vi "enumerateStaticDependencies.vi"(8 "error in (no error)":errorcluster, 11 "SMO.Example":refnum<class "SMO.TopLevel.lvclass">) -> (0 "error out":errorcluster, 2 "Static Dependencies":refnum<class "Dependency.lvclass">[](array[class]), 3 "SMO.Example out":refnum<class "SMO.TopLevel.lvclass">)   [LabVIEW 2021, in "SMO.TopLevel.lvclass"]
uses:
  SMO.TopLevel.lvclass
  SMO.TopLevel.lvclass/SMO.TopLevel.ctl
  Typedefs/Dependencies--Cluster.ctl
  SMO.A/SMO.A.lvclass
  src/SMO/SMO.lvclass
  src/Dependency/Dependency.lvclass
  C:/Repositories/SMO/src/SMO/SMO.lvclass
  C:/Repositories/SMO/tests/_test-support-SMOs/SMO.A/SMO.A.lvclass
panel:
  # "For instructions on how to use the JKI State Machine Objects, examples and video tutorials, visit:\nhttp://jki.net/state-machine-objects/\n\nJKI State Machine Objects™\nhttp://jki.net/state-machine-objects/\nCopyright (C) 2005-2015, JKI <info@jki.net>\nALL RIGHTS RESERVED"
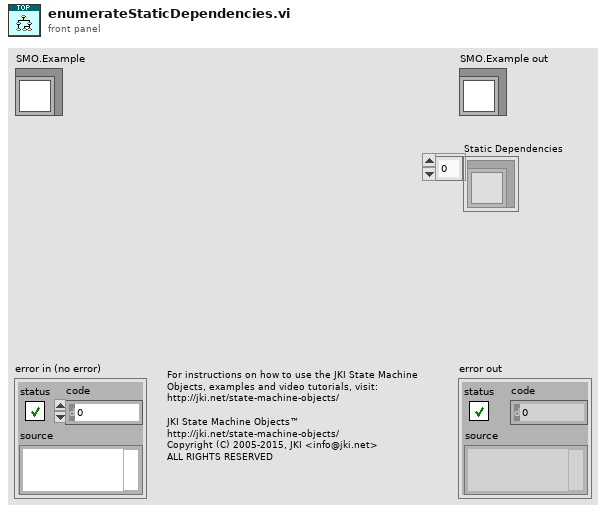
[diagram p1: front panel]
types:
  T1 = typedef "SMO.TopLevel.lvclass/Dependencies--Cluster.ctl" = cluster{"A":refnum<class "SMO.A.lvclass">, "A2":refnum<class "SMO.A.lvclass">, "A3":refnum<class "SMO.A.lvclass">, "A4":refnum<class "SMO.A.lvclass">}
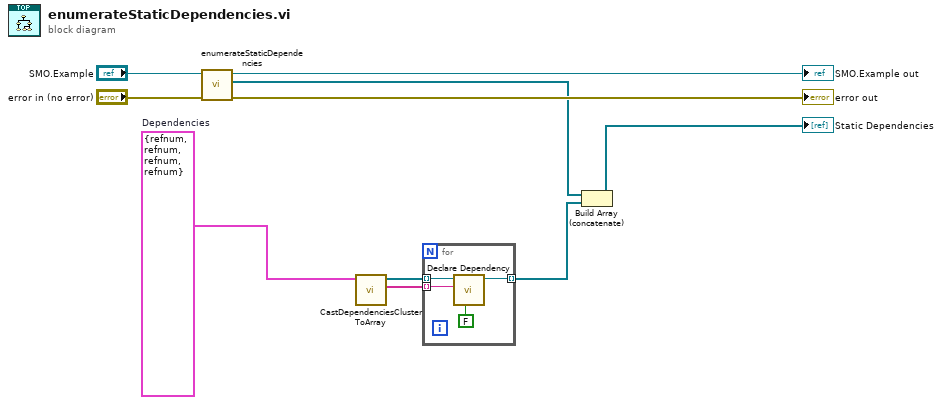
[diagram p0: block diagram]
diagram:
  w2 = T1 {"A"=refnum, "A2"=refnum, "A3"=refnum, "A4"=refnum}  # Dependencies
  n1 = call-parent "enumerateStaticDependencies.vi"("error in (no error)"="error in (no error)", "SMO"="SMO.Example") -> ("error out"=→"error out":errorcluster, "Static Dependencies"=w5:refnum<class "Dependency.lvclass">[], "SMO out"=→"SMO.Example out":refnum<class "SMO.TopLevel.lvclass">)  [unwired: 7 in]
  n2 = call "CastDependenciesClusterToArray.vi"("Dependencies Cluster"=w2) -> ("Dependencies Names"=w3:string[], "Dependencies Array"=w4:refnum<class "SMO.lvclass">[])  [unwired: 8 in, 1 out]
  n3 = for {
    tunnel: [w12] -> w1 mode=indexing
    tunnel: w4 -> [w14] mode=indexing
    tunnel: w3 -> [w13] mode=indexing
    n4 = call "Declare Dependency.vi"("Shared Resource (F)"=FALSE, "Name"=w13, "Type"=w14) -> ("Dependency out"=w12:refnum<class "Dependency.lvclass">)  [unwired: 7 in, 1 out]
  }
  n5 = Build Array (concatenate)(w5, w1) -> (→"Static Dependencies":refnum<class "Dependency.lvclass">[])
